vi "CompileDecompile.vi"() -> ()   [LabVIEW 2012]
uses:
  <vilib>/MDSplus/Library/MDSplus.lvlib
panel:
  out "Expression  out 2":string=":NUM0"
  in  "Expression":string=":NUM0"
  in  "Tree Shot":i32=-1
  in  "Tree Name":string="my_tree"
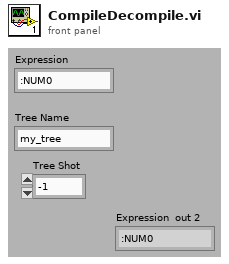
[diagram p1: front panel]
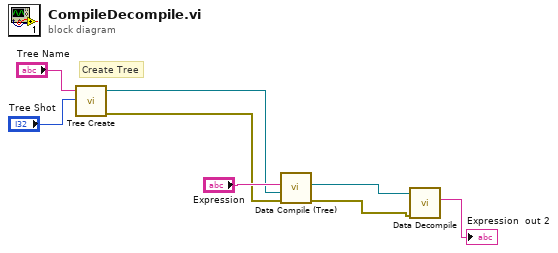
[diagram p0: block diagram]
diagram:
  # "Create Tree"
  n1 = call <vilib>:"Tree Create.vi"("Shot"="Tree Shot", "Name"="Tree Name") -> ("error out"=w2:errorcluster, "Tree DVR out"=w5:refnum<data-value>)  [unwired: 8 in]
  n2 = call <vilib>:"Data Compile (Tree).vi"("error in (no error)"=w2, "Tree in"=w5, "Expression"="Expression") -> ("error out"=w3:errorcluster, "Data out"=w1:refnum<data-value>)  [unwired: 5 in, 2 out]
  n3 = call <vilib>:"Data Decompile.vi"("error in (no error)"=w3, "Data DVR in"=w1) -> ("Expression out"=→"Expression  out 2":string)  [unwired: 7 in, 2 out]
